vi "WPI_CameraSet Enum Appearance Property.vi"(7 "Strings":string[](array[string]), 8 "error in (no error)":errorcluster, 9 "Value":i32, 10 "Property Name":string, 11 "CameraDevRef":T1) -> (0 "error out":errorcluster, 3 "CameraDevRef Out":T1)   [LabVIEW 2017]
doc: "This software is licensed. Open the labview\\readme\\WPI Robotics Library Open Source License.txt file for more information."
uses:
  <vilib>/Rock Robotics/WPI/Camera/WPI_CameraDevRef.ctl
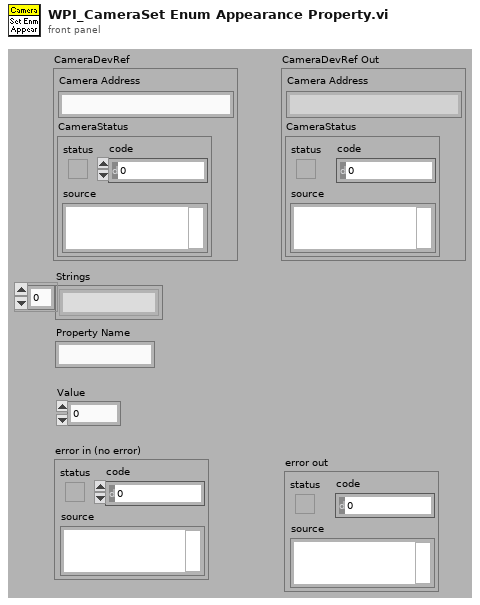
[diagram p1: front panel]
types:
  T1 = typedef "WPI_CameraDevRef.ctl" = cluster{"Camera Address":string, "CameraStatus":errorcluster}
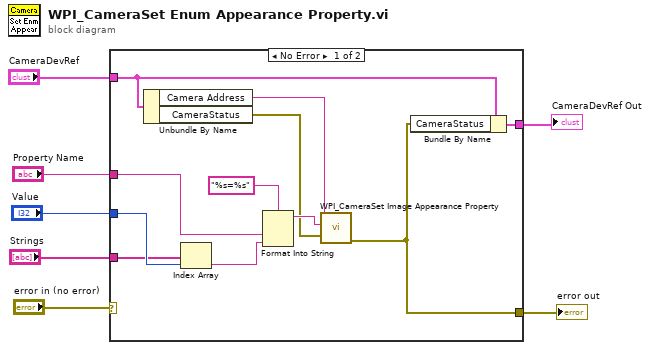
[diagram p0: block diagram]
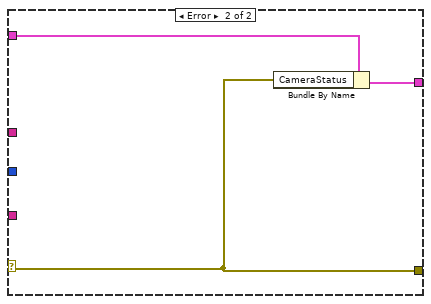
[diagram p2: hidden frame]
diagram:
  n1 = case shown="No Error" "error in (no error)" {
    selector: "error in (no error)" -> [_ w19]
    tunnel: [w18 w19] -> w7
    tunnel: [w17 w21] -> w6
    tunnel: "CameraDevRef" -> [w16 w20]
    tunnel: "Property Name" -> [w15 _]
    tunnel: "Value" -> [w12 _]
    tunnel: "Strings" -> [w9 _]
    frame No Error {
      n2 = Unbundle By Name(w16) -> ("Camera Address"=w13:string, "CameraStatus"=w8:errorcluster)
      n3 = Index Array(array=w9, index=w12) -> (element=w14:string)
      n4 = Format Into String(format string="%s=%s", w15, w14) -> (resulting string=w10:string)  [unwired: 2 in, 1 out]
      n5 = call <vilib>:"WPI_CameraSet Image Appearance Property.vi"("error in"=w8, "Prop String"=w10, "address"=w13) -> ("error out"=w18:errorcluster)  [unwired: 1 in, 7 out]
      n6 = Bundle By Name(cluster=w16, "CameraStatus"=w18) -> (w17:T1)
    }
    frame Error {
      n7 = Bundle By Name(cluster=w20, "CameraStatus"=w19) -> (w21:T1)
    }
  }
  "error out" <- w7
  "CameraDevRef Out" <- w6
